vi "Read Current Position.vi"(8 "error in (no error)":errorcluster, 11 "MotorDrive in":refnum<class "MotorDrive.lvclass">) -> (0 "error out":errorcluster, 2 "Current Position":dbl, 3 "MotorDrive out":refnum<class "MotorDrive.lvclass">)   [LabVIEW 2016, in "MotorDrive.lvclass"]
uses:
  MotorDrive.lvclass
  MotorDrive.lvclass/MotorDrive.ctl
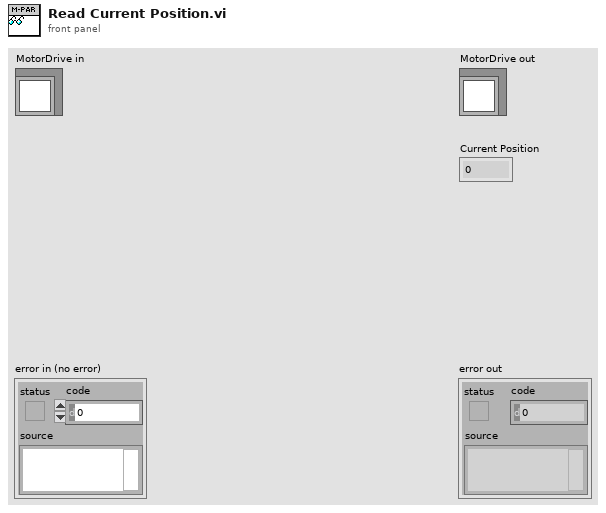
[diagram p1: front panel]
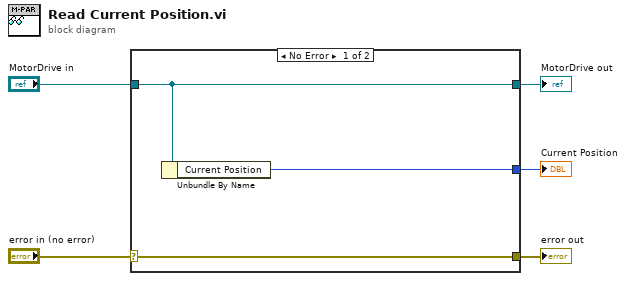
[diagram p0: block diagram]
diagram:
  n1 = case shown="No Error" "error in (no error)" {
    selector: "error in (no error)" -> [w8 w9]
    tunnel: [w8 w9] -> w4
    tunnel: [w7 w10] -> w2
    tunnel: "MotorDrive in" -> [w7 w10]
    tunnel: [w6 _] -> w1
    frame No Error {
      n2 = Unbundle By Name(w7) -> ("Current Position"=w6:i32)
    }
    frame Error {
    }
  }
  "error out" <- w4
  "MotorDrive out" <- w2
  "Current Position" <- w1
